vi "Compare Script Paths.vi"(1 "Run Instance B":refnum<class "Run Instance.lvclass">, 2 "Run Instance A":refnum<class "Run Instance.lvclass">) -> (0 "Same?":bool)   [LabVIEW 2020, in "Run Utilities.lvlib"]
doc: "Compare the script path of the two Run Instances. If the paths are the same the vi returns True"
uses:
  Run Utilities.lvlib
  Run Instance/Run Instance.lvclass
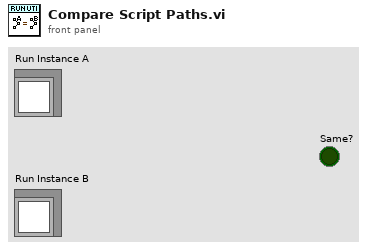
[diagram p1: front panel]
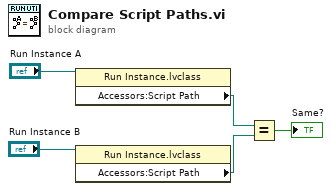
[diagram p0: block diagram]
diagram:
  n1 = property class="Run Instance.lvclass"(reference="Run Instance A") -> ("Accessors:Script Path"=w3:path)  [unwired: 1 in, 2 out]
  n2 = property class="Run Instance.lvclass"(reference="Run Instance B") -> ("Accessors:Script Path"=w1:path)  [unwired: 1 in, 2 out]
  n3 = Equal?(x=w3, y=w1) -> (x = y?=→"Same?":bool)
